vi "Get Device Status.vi"(8 "error in (no error)":errorcluster, 11 "NRT8000 in":refnum<class "NRT8000.lvclass">) -> (0 "error out":errorcluster, 2 "Status":string, 3 "NRT8000 out":refnum<class "NRT8000.lvclass">)   [LabVIEW 2018, in "NRT8000.lvlib" / "NRT8000.lvclass"]
uses:
  NRT8000.lvclass
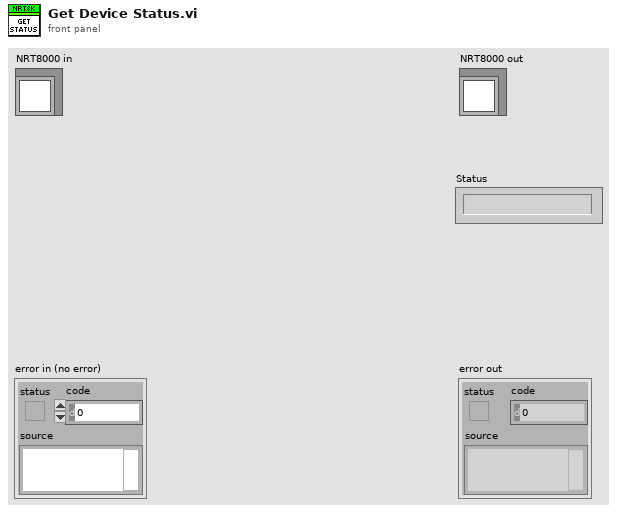
[diagram p1: front panel]
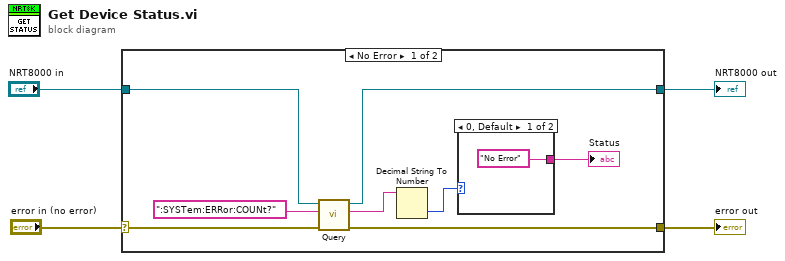
[diagram p0: block diagram]
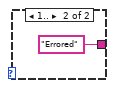
[diagram p2: hidden frame]
diagram:
  n1 = case shown="No Error" "error in (no error)" {
    selector: "error in (no error)" -> [w10 w16]
    tunnel: [w8 w16] -> w3
    tunnel: [w11 w15] -> w2
    tunnel: "NRT8000 in" -> [w12 w15]
    frame No Error {
      n2 = call "Query.vi"("error in (no error)"=w10, "Cmd"=":SYSTem:ERRor:COUNt?", "NRT8000 in"=w12) -> ("error out"=w8:errorcluster, "Rsp"=w7:string, "NRT8000 out"=w11:refnum<class "NRT8000.lvclass">)  [unwired: 6 in]
      n3 = Decimal String To Number(string=w7) -> (number=w6:i32)  [unwired: 2 in, 1 out]
      n4 = case shown="0, Default" w6 {
        tunnel: ["No Error" ("String") "Errored"] -> w5
        frame 0, Default {
        }
        frame 1.. {
        }
      }
      "Status" <- w5
    }
    frame Error {
    }
  }
  "error out" <- w3
  "NRT8000 out" <- w2
